vi "dmm_measurement.vi"(4 "Session Name":string="SampleDMM") -> (0 "error out":errorcluster, 1 "reading":dbl format="%^.2e")   [LabVIEW 2011]
doc: "This VI gets the session that Session Name specifies and converts it into an IVI instrument handle\nbefore calling an IviDmm class driver method to make a measurement. It then closes the reference\nto the existing Instrument Session that Get Instrument Session.vi returned."
uses:
  <vilib>/addons/TestStand/_SMUtility.llb/Session Manager - Get Instrument Session (32-bit).vi
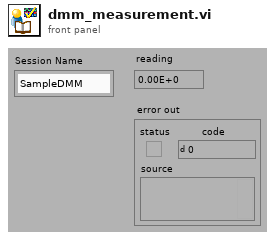
[diagram p1: front panel]
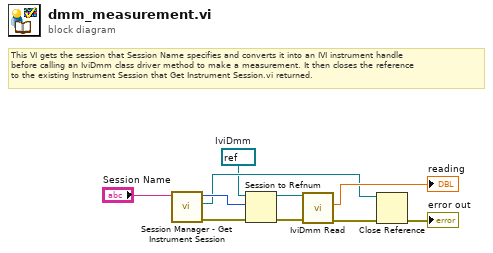
[diagram p0: block diagram]
diagram:
  w2 = refnum<k15> refnum  # IviDmm
  # "This VI gets the session that Session Name specifies and converts it into an IVI instrument handle\nbefore calling an IviDmm class driver method to make a measurement. It then closes the reference\nto the existing Instrument Session that Get Instrument Session.vi returned."
  n1 = call-poly <vilib>:"Session Manager - Get Instrument Session.vi"("Session Name"="Session Name") -> ("error out"=w9:errorcluster, "Instrument Session"=w3:refnum<k7>, "Driver Handle"=w10:u32)  [unwired: 8 in]
  n2 = Session to Refnum(4:w9, 6:w10, 7:w2) -> (0:w8:errorcluster, 3:w7:refnum<k15>)
  n3 = call <vilib>:"IviDmm Read.vi"("error in (no error)"=w8, "instrument handle"=w7) -> ("error out"=w5:errorcluster, "reading"=→"reading":dbl)  [unwired: 7 in, 1 out]
  n4 = Close Reference(reference=w3, error in (no error)=w5) -> (error out=→"error out":errorcluster)
